vi "Roi_test.vi"() -> ()   [LabVIEW 2021]
panel:
  in  "stop":bool
  out "Image":T1(plugin-control)
  in  "input image":path
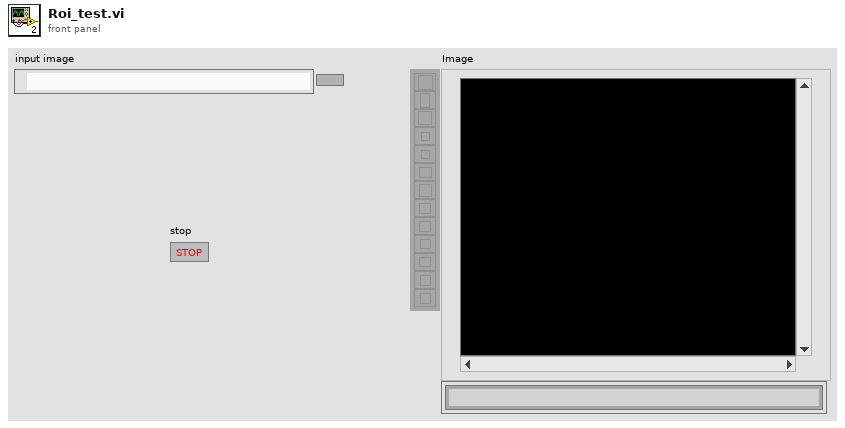
[diagram p1: front panel]
types:
  T1 = typedef "IMAQ Image.ctl" = refnum<image>
  T2 = cluster{"Desired Font (Application)":enum16{"User-specified Font", "Application Font", "System Font", "Dialog Font"}, "[User-specified Font]":cluster{"Font Name":string, "Size":i16, "Strikeout?":bool, "Italic?":bool, "Underline?":bool, "Outline?":bool, "Shadow?":bool, "Bold?":bool, "Rotation Angle":dbl}, "Horizontal Alignment":i16, "Vertical Alignment":i16}
  T3 = cluster{"Global Rectangle":i32[], "Contours":cluster{"Contour Type":u32, "ROI Type":u32, "Points":i32[]}[]}
  T4 = cluster{"Contour Type":u32, "ROI Type":u32, "Points":i32[]}[]
  T5 = cluster{"Contour Type":u32, "ROI Type":u32, "Points":i32[]}
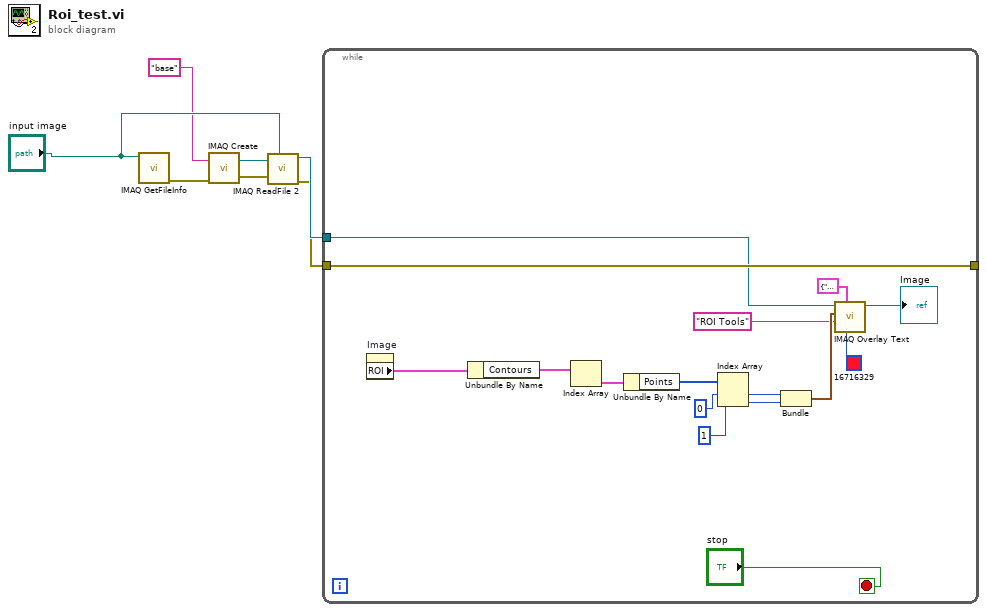
[diagram p0: block diagram]
diagram:
  n1 = call "IMAQ GetFileInfo"("File Path"="input image") -> ("error out"=w7:errorcluster)  [unwired: 4 in, 6 out]
  n2 = call "IMAQ Create"("Image Name"="base", "error in (no error)"=w7) -> ("New Image"=w6:T1, "error out"=w5:errorcluster)  [unwired: 3 in]
  n3 = call "IMAQ ReadFile 2"("File Path"="input image", "error in (no error)"=w5, "Image"=w6) -> ("error out"=w3:errorcluster, "Image Out"=w4:T1)  [unwired: 4 in, 3 out]
  n4 = while {
    tunnel: w4 -> [w11]
    tunnel: w3 -> [w23]
    tunnel: [w23] -> _
    stop <- "stop" stop-if-true
    n5 = property on="Image" class="ImageControl"() -> ("ROI"=w21:T3)  [unwired: 2 in, 2 out]
    n6 = Unbundle By Name(w21) -> ("Contours"=w20:T4)
    n7 = Index Array(array=w20) -> (element=w19:T5)  [unwired: 1 in]
    n8 = Unbundle By Name(w19) -> ("Points"=w18:i32[])
    n9 = Index Array(array=w18, index #1=0 ("index"), index #2=1 ("index")) -> (element #1=w14:i32, element #2=w15:i32)
    n10 = Bundle(w14, w15) -> (w13:cluster{i32, i32})  [unwired: 1 in]
    n11 = call "IMAQ Overlay Text"("Text Color (black)"=u32 16716329 ("BG Color (Transparent)"), "Font, Size & Style"=T2 {"Desired Font (Application)"=enum."Application Font", "[User-specified Font]"={"Font Name"="", "Size"=40, "Strikeout?"=FALSE, "Italic?"=FALSE, "Underline?"=FALSE, "Outline?"=FALSE, "Shadow?"=FALSE, "Bold?"=FALSE, "Rotation Angle"=0.0}, "Horizontal Alignment"=0, "Vertical Alignment"=0}, "String"="ROI Tools", "Origin"=w13, "Image"=w11) -> ("Image Out"=→"Image":T1)  [unwired: 5 in, 1 out]
  }
